vi "Driver Stick.vi"() -> (10 "String 4":string, 12 "String 3":string, 13 "String 8":string, 14 "String 2":string, 15 "String 9":string, 16 "String":string, 17 "String 10":string, 18 "String 16":string, 19 "String 11":string, 20 "String 15":string, 21 "String 5":string, 22 "String 14":string, 23 "String 6":string, 24 "String 13":string, 25 "String 7":string, 26 "String 12":string)   [LabVIEW 2015]
uses:
  <vilib>/Rock Robotics/Network Tables/NT Read Boolean.vi
  <vilib>/Rock Robotics/Network Tables/NT Read Number.vi
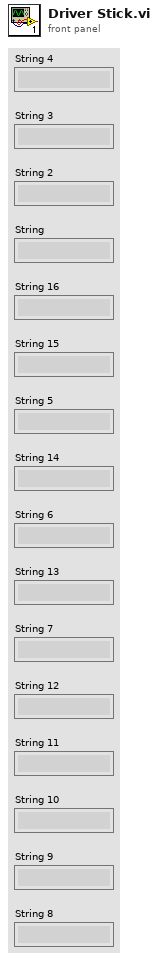
[diagram p1: front panel]
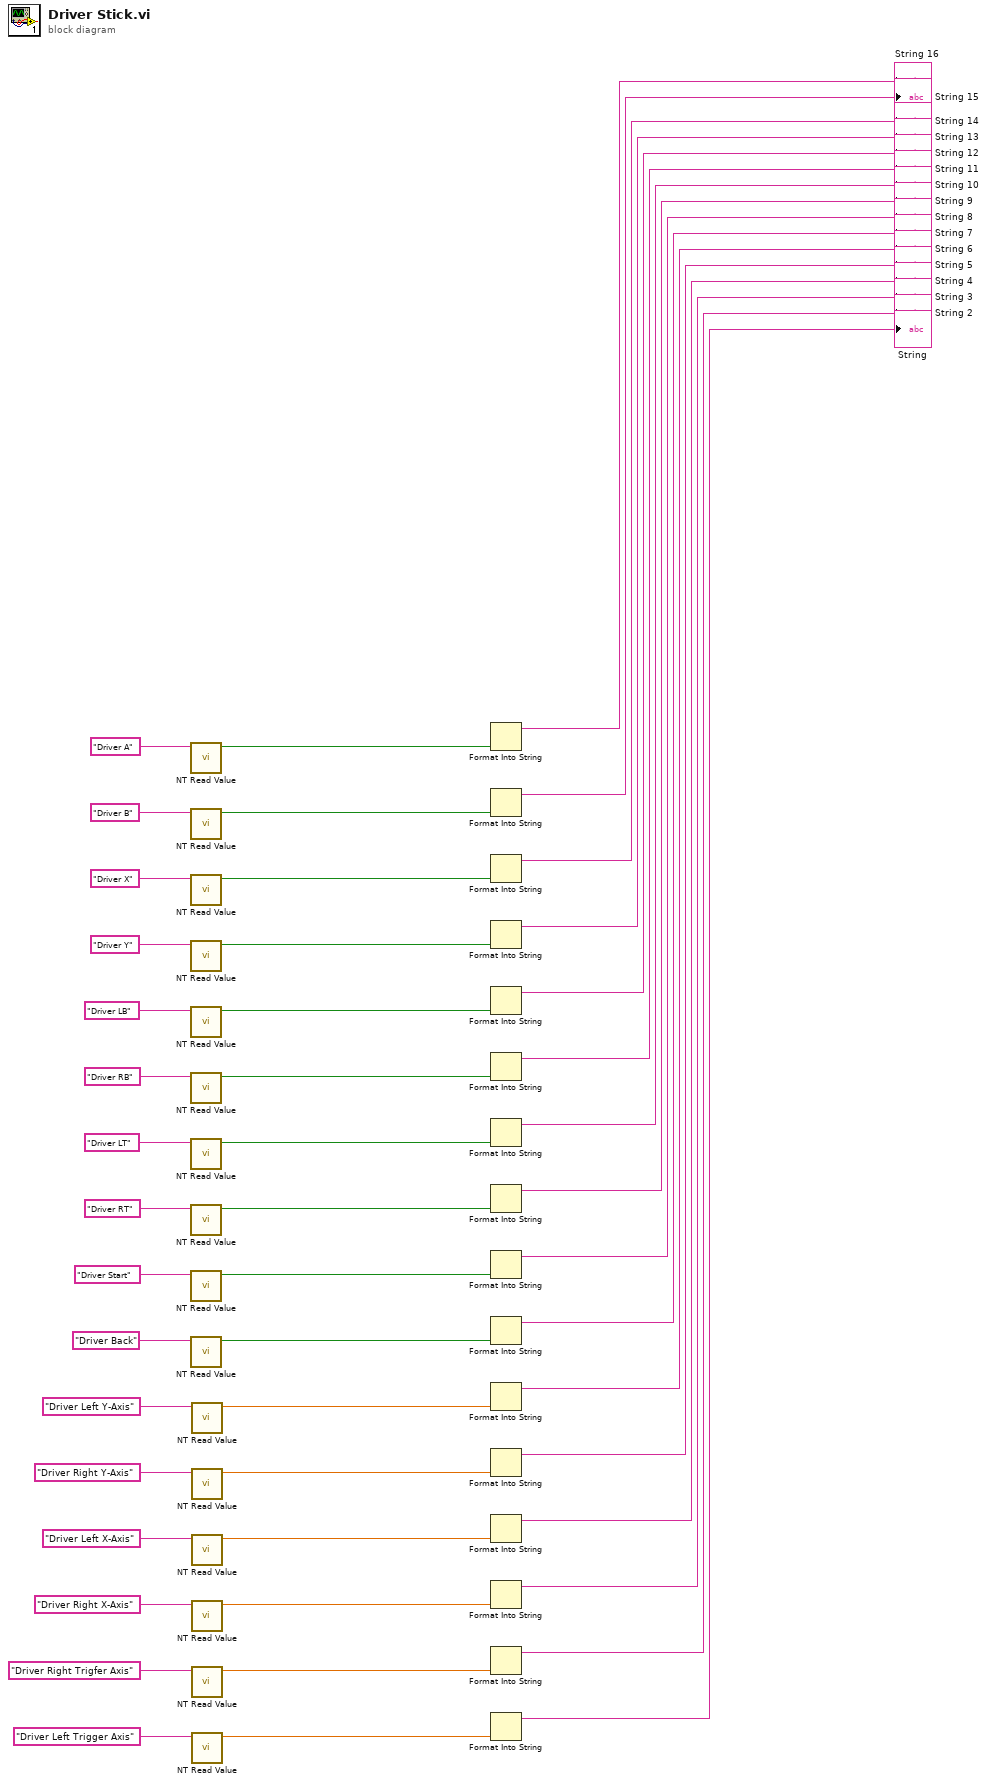
[diagram p0: block diagram]
diagram:
  n1 = call-poly <vilib>:"NT Read Value.vi"("Name"="Driver A") -> ("Boolean"=w3:bool)  [unwired: 9 in, 1 out]
  n2 = call-poly <vilib>:"NT Read Value.vi"("Name"="Driver B") -> ("Boolean"=w1:bool)  [unwired: 9 in, 1 out]
  n3 = call-poly <vilib>:"NT Read Value.vi"("Name"="Driver X") -> ("Boolean"=w7:bool)  [unwired: 9 in, 1 out]
  n4 = call-poly <vilib>:"NT Read Value.vi"("Name"="Driver Y") -> ("Boolean"=w9:bool)  [unwired: 9 in, 1 out]
  n5 = call-poly <vilib>:"NT Read Value.vi"("Name"="Driver LB") -> ("Boolean"=w11:bool)  [unwired: 9 in, 1 out]
  n6 = call-poly <vilib>:"NT Read Value.vi"("Name"="Driver RB") -> ("Boolean"=w13:bool)  [unwired: 9 in, 1 out]
  n7 = call-poly <vilib>:"NT Read Value.vi"("Name"="Driver LT") -> ("Boolean"=w19:bool)  [unwired: 9 in, 1 out]
  n8 = call-poly <vilib>:"NT Read Value.vi"("Name"="Driver RT") -> ("Boolean"=w21:bool)  [unwired: 9 in, 1 out]
  n9 = call-poly <vilib>:"NT Read Value.vi"("Name"="Driver Start") -> ("Boolean"=w23:bool)  [unwired: 9 in, 1 out]
  n10 = call-poly <vilib>:"NT Read Value.vi"("Name"="Driver Back") -> ("Boolean"=w25:bool)  [unwired: 9 in, 1 out]
  n11 = call-poly <vilib>:"NT Read Value.vi"("Name"="Driver Left Y-Axis") -> ("Numeric"=w31:dbl)  [unwired: 9 in, 1 out]
  n12 = call-poly <vilib>:"NT Read Value.vi"("Name"="Driver Right Y-Axis") -> ("Numeric"=w34:dbl)  [unwired: 9 in, 1 out]
  n13 = call-poly <vilib>:"NT Read Value.vi"("Name"="Driver Left X-Axis") -> ("Numeric"=w37:dbl)  [unwired: 9 in, 1 out]
  n14 = call-poly <vilib>:"NT Read Value.vi"("Name"="Driver Right X-Axis") -> ("Numeric"=w39:dbl)  [unwired: 9 in, 1 out]
  n15 = call-poly <vilib>:"NT Read Value.vi"("Name"="Driver Right Trigfer Axis") -> ("Numeric"=w43:dbl)  [unwired: 9 in, 1 out]
  n16 = call-poly <vilib>:"NT Read Value.vi"("Name"="Driver Left Trigger Axis") -> ("Numeric"=w45:dbl)  [unwired: 9 in, 1 out]
  n17 = Format Into String(w3) -> (resulting string=→"String 16":string)  [unwired: 3 in, 1 out]
  n18 = Format Into String(w1) -> (resulting string=→"String 15":string)  [unwired: 3 in, 1 out]
  n19 = Format Into String(w7) -> (resulting string=→"String 14":string)  [unwired: 3 in, 1 out]
  n20 = Format Into String(w9) -> (resulting string=→"String 13":string)  [unwired: 3 in, 1 out]
  n21 = Format Into String(w11) -> (resulting string=→"String 12":string)  [unwired: 3 in, 1 out]
  n22 = Format Into String(w13) -> (resulting string=→"String 11":string)  [unwired: 3 in, 1 out]
  n23 = Format Into String(w19) -> (resulting string=→"String 10":string)  [unwired: 3 in, 1 out]
  n24 = Format Into String(w21) -> (resulting string=→"String 9":string)  [unwired: 3 in, 1 out]
  n25 = Format Into String(w23) -> (resulting string=→"String 8":string)  [unwired: 3 in, 1 out]
  n26 = Format Into String(w25) -> (resulting string=→"String 7":string)  [unwired: 3 in, 1 out]
  n27 = Format Into String(w31) -> (resulting string=→"String 6":string)  [unwired: 3 in, 1 out]
  n28 = Format Into String(w34) -> (resulting string=→"String 5":string)  [unwired: 3 in, 1 out]
  n29 = Format Into String(w37) -> (resulting string=→"String 4":string)  [unwired: 3 in, 1 out]
  n30 = Format Into String(w39) -> (resulting string=→"String 3":string)  [unwired: 3 in, 1 out]
  n31 = Format Into String(w43) -> (resulting string=→"String 2":string)  [unwired: 3 in, 1 out]
  n32 = Format Into String(w45) -> (resulting string=→"String":string)  [unwired: 3 in, 1 out]
